vi "3.vi"() -> ()   [LabVIEW 2019]
panel:
  out "Iteration Count":dbl
  in  "Stop":bool
  out "Output":dbl
  in  "Operation":enum16{"Add", "Subtract", "Multiply", "Divide"}(ring)
  in  "B":dbl
  in  "A":dbl
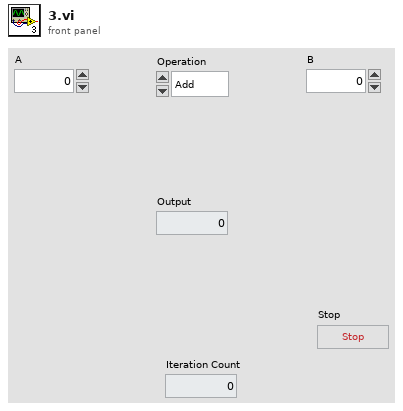
[diagram p1: front panel]
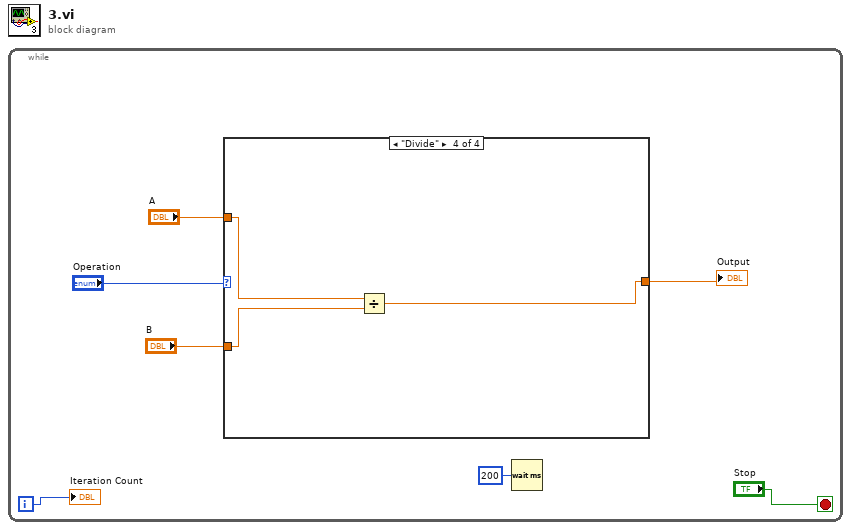
[diagram p0: block diagram]
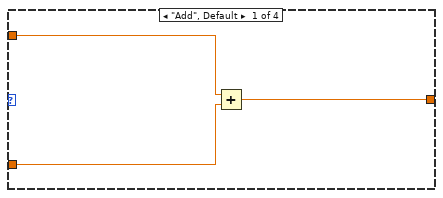
[diagram p2: hidden frame]
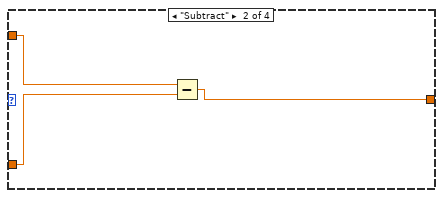
[diagram p3: hidden frame]
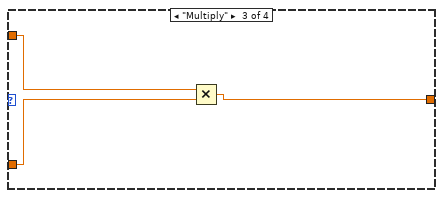
[diagram p4: hidden frame]
diagram:
  n1 = while {
    i -> [w2]
    stop <- "Stop" stop-if-true
    n2 = case shown="\"Divide\"" "Operation" {
      tunnel: "A" -> [w10 w13 w16 w19]
      tunnel: "B" -> [w9 w12 w15 w18]
      tunnel: [w8 w11 w14 w17] -> w4
      frame "Add", Default {
        n3 = Add(x=w10, y=w9) -> (x+y=w8:dbl)
      }
      frame "Subtract" {
        n4 = Subtract(x=w13, y=w12) -> (x-y=w11:dbl)
      }
      frame "Multiply" {
        n5 = Multiply(x=w16, y=w15) -> (x*y=w14:dbl)
      }
      frame "Divide" {
        n6 = Divide(x=w19, y=w18) -> (x/y=w17:dbl)
      }
    }
    "Output" <- w4
    n7 = Wait (ms)(milliseconds to wait=u32 200) -> ()  [unwired: 1 out]
    "Iteration Count" <- w2
  }
